vi "Read Builder Configuration.vi"(8 "error in (no error)":errorcluster, 11 "Builder in":refnum<class "Builder.lvclass">) -> (0 "error out":errorcluster, 3 "Builder out":refnum<class "Builder.lvclass">)   [LabVIEW 2019, in "Builder.lvclass"]
doc: "Read the configuration for the Builder. This is specific to the company and author, not the library being built. It is anticipated that these values can be found in the same repository as this code, rather than in the built code."
uses:
  Builder.lvclass
  Builder.lvclass/Builder.ctl
  <vilib>/Utility/config.llb/Read Key (String).vi
  <vilib>/Utility/config.llb/NI_LVConfig.lvlib
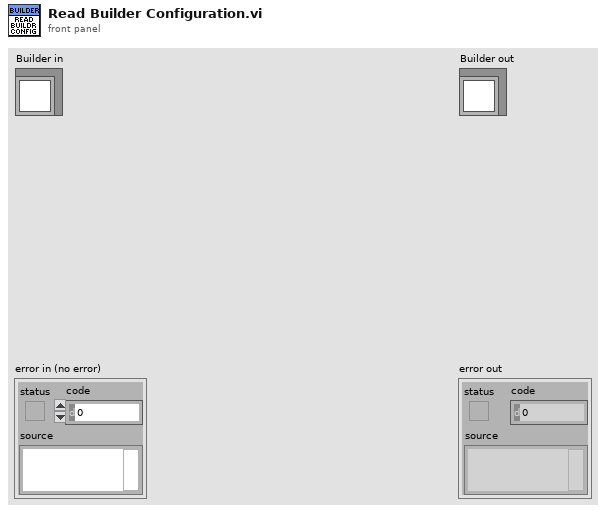
[diagram p1: front panel]
types:
  T1 = typedef "NI_LVConfig.lvlib/Config Data RefNum.ctl" = refnum<k1>
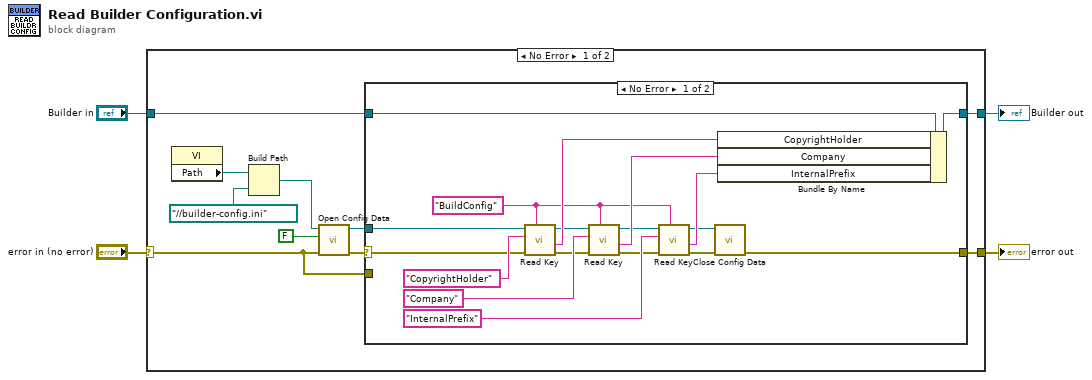
[diagram p0: block diagram]
diagram:
  n1 = case shown="No Error" "error in (no error)" {
    selector: "error in (no error)" -> [w8 w36]
    tunnel: [w7 w36] -> w3
    tunnel: [w6 w35] -> w1
    tunnel: "Builder in" -> [w5 w35]
    frame No Error {
      n2 = property class="VI"() -> ("Path"=w11:path)  [unwired: 2 in, 2 out]
      n3 = Build Path(base path=w11, name or relative path=path "../../builder-config.ini") -> (appended path=w9:path)
      n4 = call <vilib>:"Open Config Data.vi"("error in (no error)"=w8, "create file if necessary (T)"=FALSE, "configuration file path"=w9) -> ("error out"=w13:errorcluster, "refnum"=w14:T1)  [unwired: 6 in, 1 out]
      n5 = case shown="No Error" w13 {
        selector: w13 -> [w25 _]
        tunnel: w14 -> [w26 _]
        tunnel: [w18 w34] -> w7
        tunnel: w8 -> [_ w34]
        tunnel: w5 -> [w16 w33]
        tunnel: [w15 w33] -> w6
        frame No Error {
          w17 = "BuildConfig" ("section")
          n6 = call-poly <vilib>:"Read Key.vi"("section"=w17, "error in (no error)"=w25, "key"="CopyrightHolder", "refnum"=w26) -> ("error out"=w23:errorcluster, "value"=w29:string, "refnum out"=w24:T1)  [unwired: 4 in, 1 out]
          n7 = call-poly <vilib>:"Read Key.vi"("section"=w17, "error in (no error)"=w23, "key"="Company", "refnum"=w24) -> ("error out"=w21:errorcluster, "value"=w28:string, "refnum out"=w22:T1)  [unwired: 4 in, 1 out]
          n8 = call-poly <vilib>:"Read Key.vi"("section"=w17, "error in (no error)"=w21, "key"="InternalPrefix", "refnum"=w22) -> ("error out"=w19:errorcluster, "value"=w27:string, "refnum out"=w20:T1)  [unwired: 4 in, 1 out]
          n9 = call <vilib>:"Close Config Data.vi"("error in (no error)"=w19, "refnum"=w20) -> ("error out"=w18:errorcluster)  [unwired: 8 in, 1 out]
          n10 = Bundle By Name(cluster=w16, "CopyrightHolder"=w29, "Company"=w28, "InternalPrefix"=w27) -> (w15:refnum<class "Builder.lvclass">)
        }
        frame Error {
        }
      }
    }
    frame Error {
    }
  }
  "error out" <- w3
  "Builder out" <- w1
